vi "Picolog Get temperature.vi"(6 "Units":T2, 7 "Fill Missing Points":T1 items=["QNaN", "Previous"], 8 "Error In":errorcluster, 9 "Channel":i16, 10 "Buffer length":i32=128, 11 "Instrument Handle In":i16) -> (0 "Error Out":errorcluster, 1 "Temperature":sgl[](array[numeric]), 2 "Time [s]":dbl[](array[numeric]), 3 "Instrument Handle Out":i16, 4 "Overflow":i16)   [LabVIEW 2017]
uses:
  Controls/Temperature Units.ctl
  Controls/Fill Missing.ctl
  usbtc08.dll
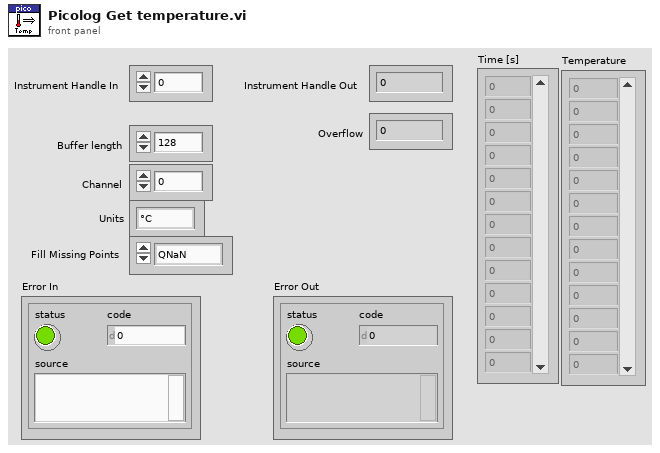
[diagram p1: front panel]
types:
  T1 = typedef "Fill Missing.ctl" = i16
  T2 = typedef "Temperature Units.ctl" = enum16{"°C", "°F", "K", "°R"}
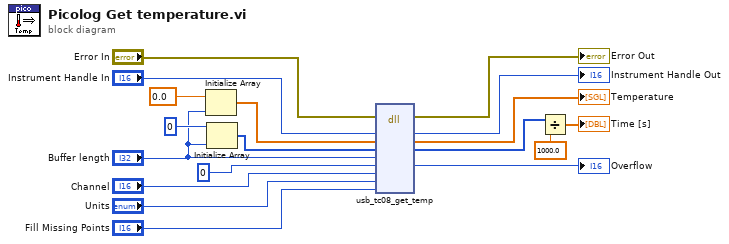
[diagram p0: block diagram]
diagram:
  n1 = Initialize Array(sgl 0.0, "Buffer length") -> (w13:sgl[])
  n2 = Initialize Array(0 ("Numeric Control"), "Buffer length") -> (w8:i32[])
  n3 = dll-call lib="usbtc08.dll" fn="usb_tc08_get_temp"(error in="Error In", "handle"="Instrument Handle In", "temp_buffer"=w13, "times_ms_buffer"=w8, "buffer length"="Buffer length", "overflow"=i16 0, "channel"="Channel", "units"="Units", "fill_missing"="Fill Missing Points") -> (error out=→"Error Out":errorcluster, "handle"=→"Instrument Handle Out":i16, "temp_buffer"=→"Temperature":sgl[], "times_ms_buffer"=w5:i32[], "overflow"=→"Overflow":i16)  [unwired: 7 in, 1 out]
  n4 = Divide(x=w5, y=1000.0) -> (x/y=→"Time [s]":dbl[])
